vi "delete.vi"(8 "error in (no error)":errorcluster, 9 "range":i32=1 min=1, 10 "start index":i32 min=0, 11 "ImageCollection in":refnum<class "ImageCollection.lvclass">) -> (0 "error out":errorcluster, 3 "ImageCollection out":refnum<class "ImageCollection.lvclass">)   [LabVIEW 2010, in "ImageCollection.lvclass"]
uses:
  ImageCollection.lvclass
  Image/Image/Image.lvclass
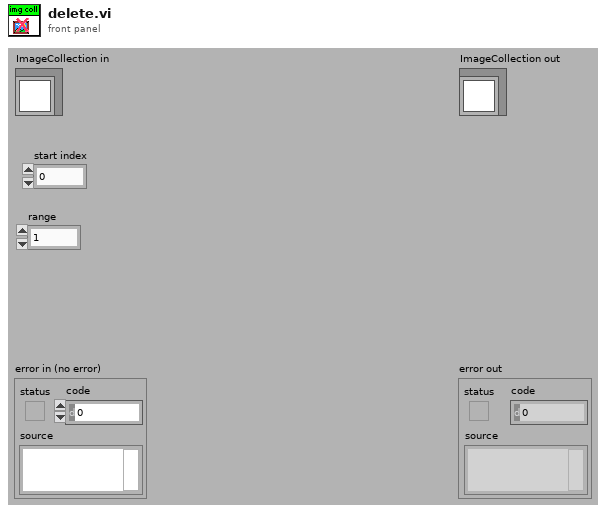
[diagram p1: front panel]
types:
  T1 = typedef "ImageCollection.lvclass/storage_mode_enum.ctl" = enum16{"RAM", "single files", "multipage TIFF (read-only)"}
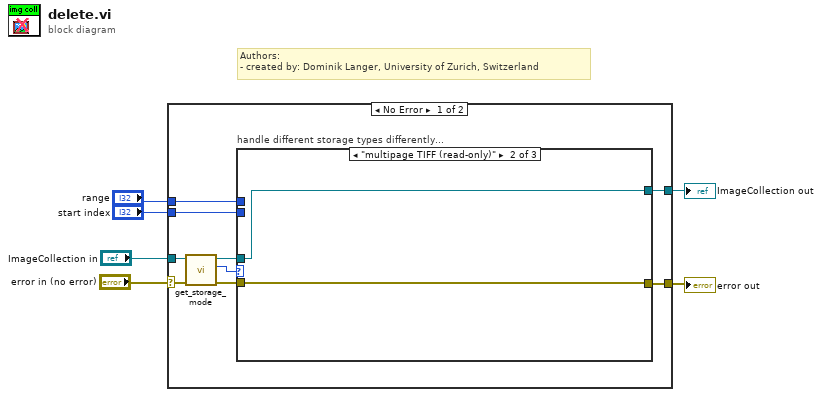
[diagram p0: block diagram]
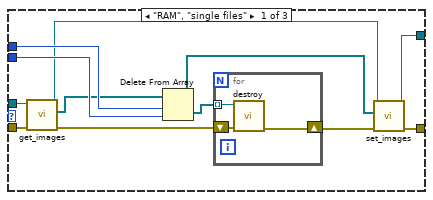
[diagram p2: hidden frame]
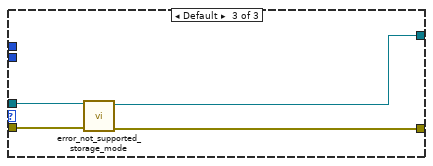
[diagram p3: hidden frame]
diagram:
  # "Authors: \n- created by: Dominik Langer, University of Zurich, Switzerland"
  n1 = case shown="No Error" "error in (no error)" {
    selector: "error in (no error)" -> [w11 w38]
    tunnel: [w14 w38] -> w5
    tunnel: [w15 w37] -> w3
    tunnel: "ImageCollection in" -> [w9 w37]
    tunnel: "start index" -> [w13 _]
    tunnel: "range" -> [w12 _]
    frame No Error {
      n2 = call-dynamic "get_storage_mode.vi"("error in (no error)"=w11, "ImageCollection.lvclass in"=w9) -> ("error out"=w10:errorcluster, "storage type"=w8:T1, "ImageCollection.lvclass out"=w7:refnum<class "ImageCollection.lvclass">)  [unwired: 7 out]
      n3 = case "handle different storage types differently..." shown="\"multipage TIFF (read-only)\"" w8 {
        tunnel: [w22 w31 w34] -> w15
        tunnel: [w23 w32 w33] -> w14
        tunnel: w13 -> [w25 _ _]
        tunnel: w12 -> [w26 _ _]
        tunnel: w10 -> [w20 w32 w36]
        tunnel: w7 -> [w19 w31 w35]
        frame "RAM", "single files" {
          n4 = call-dynamic "get_images.vi"("error in (no error)"=w20, "ImageCollection.lvclass in"=w19) -> ("error out"=w18:errorcluster, "images"=w16:refnum<class "Image.lvclass">[], "ImageCollection.lvclass out"=w17:refnum<class "ImageCollection.lvclass">)  [unwired: 7 out]
          n5 = Delete From Array(array=w16, length=w26, index=w25) -> (deleted portion=w27:refnum<class "Image.lvclass">[], array with subset deleted=w21:refnum<class "Image.lvclass">[])
          n6 = for {
            tunnel: w27 -> [w30] mode=indexing
            shift-right: [w28] -> w24
            shift-left: w18 -> [w29]
            n7 = call-dynamic "destroy.vi"("error in (no error)"=w29, "Image in"=w30) -> ("error out"=w28:errorcluster)  [unwired: 9 out]
          }
          n8 = call-dynamic "set_images.vi"("error in (no error)"=w24, "images"=w21, "ImageCollection.lvclass in"=w17) -> ("error out"=w23:errorcluster, "ImageCollection.lvclass out"=w22:refnum<class "ImageCollection.lvclass">)  [unwired: 7 out]
        }
        frame "multipage TIFF (read-only)" {
        }
        frame Default {
          n9 = call-dynamic "error_not_supported_storage_mode.vi"("error in (no error)"=w36, "ImageCollection in"=w35) -> ("error out"=w33:errorcluster, "ImageCollection out"=w34:refnum<class "ImageCollection.lvclass">)  [unwired: 8 out]
        }
      }
    }
    frame Error {
    }
  }
  "error out" <- w5
  "ImageCollection out" <- w3
